vi "10-Tap 8-bit Camera with DRAM (FPGA).vi"() -> ()   [LabVIEW 2013]
doc: "This is the FPGA VI for the 10-Tap 8-Bit Camera with DRAM example. This example demonstrates how to acquire images from a 10-tap, 8-bit, extended configuration, Camera Link camera and transfer the images to the host. This example supports area scan and line scan cameras for both continuous and finite acquisitions.\n\nThis example also demonstrates the use of DRAM as a frame buffer for very high speed acquisitions. Data packing and flow-control are also employed to maximize use of the available DRAM and FIFOs in terms of both memory space and performance.\n\nAdditionally, the example demonstrates the serial server, which allows third-party camera configuration utilities to communicate with the camera using the Camera Link serial interface while this VI is running."
uses:
  Common/CL Signal Mapping.ctl
  Common/CL Configuration.ctl
  FPGA/Sector/Accumulate/Sector Parameter Cluster.ctl
  <vilib>/Platform/TimedLoop/XDataNode/timing_clust.ctl
  <vilib>/Platform/TimedLoop/XDataNode/nitl_modes.ctl
  <vilib>/Platform/TimedLoop/XDataNode/wakeup.ctl
  <vilib>/rvi/Emulation/niFpgaSctlEmulationGetInTimedLoop.vi
  <vilib>/rvi/Emulation/niFpgaEmulationReportErrorSimple.vi
  <vilib>/rvi/Emulation/niFpgaGetClockAttributes.vi
  <vilib>/rvi/Emulation/niFpgaCriticalErrorInLSC.vi
  <vilib>/rvi/eio/common/nirviEmuTemplateMethod_errors.vi
  FPGA/Globals/Wing Square Wave Frequency Global.vi
  <vilib>/rvi/interface/RandomDataEmulation/nirviRandomDataFPGAFIFO.vi
  <vilib>/rvi/interface/RandomDataEmulation/niFpgaRandomDataHandleErrors.vi
  <vilib>/rvi/FIFO/Fifo_Resource/nirvififoEmulationWriteFpgaImpl.vi
  <vilib>/rvi/DataTransferAndStorage/Container/Common/niFpgaContainerGetUniqueNameForEmu.vi
  <vilib>/rvi/FIFO/Fifo_Resource/nirvififoEmulationGetNumberOfElementsToReadFpgaImpl.vi
  <vilib>/rvi/FIFO/Fifo_Resource/nirvififoEmulationReadFpgaImpl.vi
  <vilib>/rvi/FIFO/Fifo_Resource/nirvififoEmulationGetNumberOfElementsToWriteFpgaImpl.vi
  <vilib>/rvi/Emulation/niFpgaProcessEmulError.vi
  FPGA/Globals/Sector Parameter Global.vi
  FPGA/Globals/Accumulated Sector Intensity.vi
  FPGA/Globals/Pixel Location Global.vi
  <vilib>/Platform/TimedLoop/XDataNode/XDataNode.xnode
  <vilib>/eio/EIONode/EIONode.xnode
  <vilib>/rvi/DataTransferAndStorage/Container/XNode/niFpgaContainer.xnode
  <vilib>/rvi/interface/RandomDataEmulation/nirviRandomDataFpgaReadWriteTemplate.vi
  <vilib>/rvi/FIFO/Fifo_Resource/nirvififoEmulationWrite.vi
  <vilib>/rvi/FIFO/Fifo_Resource/nirvififoEmulationGetNumberOfElementsToRead.vi
  <vilib>/rvi/FIFO/Fifo_Resource/nirvififoEmulationRead.vi
  <vilib>/rvi/FIFO/Fifo_Resource/nirvififoEmulationGetNumberOfElementsToWrite.vi
  <vilib>/Platform/TimedLoop/XDataNode/XDNodeRunTimeDep.lvlib
  Common/CL Data to Pixels/10 Tap 8-Bit.vi
  FPGA/10-Tap Data/10-Tap Conversion Enum.ctl
panel:
  in  "[Average BG Intensity]":u8[](array[numeric])=[0, 0, 0, 0, 0, 0, 0, 0, 0, 0, 0, 0, 0, 0, 0, 0, 0, 0, 0, 0, 0, 0, 0, 0, 0, 0, 0, 0, 0, 0, 0, 0]
  in  "Sector Threshold":u8
  in  "# of Frames to Average":u8
  in  "Sector Parameters Right":T1={"Start Angle"=0.0, "End Angle"=0.4708251953125, "Inner Radius"=309, "Outter Radius"=405, "Hinge X"=685, "Hinge Y"=527, "NumWingSectors"=8}
  in  "Sector Parameters Left":T1={"Start Angle"=0.65740966796875, "End Angle"=0.99468994140625, "Inner Radius"=309, "Outter Radius"=405, "Hinge X"=464, "Hinge Y"=534, "NumWingSectors"=8}
  in  "Sim":bool=TRUE
  in  "CL Config.Configuration":T2=enum."Full"
  in  "CL Config.Signal Mapping":T3=enum."Basler 10-tap"
  in  "CL Config.Line Scan":bool
  in  "CL Config.DVAL Active High":bool=TRUE
  in  "CL Config.LVAL Active High":bool=TRUE
  in  "CL Config.FVAL Active High":bool=TRUE
  in  "CL Config.Spare Active High":bool=TRUE
  in  "Acq Control.Line Scan Height":u32
  in  "Acq Control.Frames To Acq":u32
  in  "Acq Control.Acquire":bool
  in  "Acq Control.Cancel Acq":bool
  in  "Acq Control.Ignore DVAL":bool
  in  "Acq Control.Initialize":bool
  out "Acq Status.Acq In Progress":bool
  out "Acq Status.Clocks Per Line":u32
  out "Acq Status.Frames Acq'd":u32
  out "Acq Status.Lines Per Frame":u32
  out "Acq Status.DMA Write Timeout":bool
  out "Acq Status.Initialized":bool
  in  "UART.Baud Rate":u8
  in  "UART.Transmit":bool
  in  "UART.Tx Data":u8[](array[numeric])=[0, 0, 0, 0, 0, 0, 0, 0, 0, 0] format="%02x"
  in  "UART.Set Baud Rate":bool
  in  "UART.Byte Mode":bool=TRUE
  out "UART.Rx Ready":bool
  out "UART.Break Indicator":bool
  out "UART.Framing Error":bool
  out "UART.Overrun Error":bool
  out "UART.Tx Ready":bool
  out "UART.Rx Data":u8 format="%02x"
  in  "UART.Receive":bool
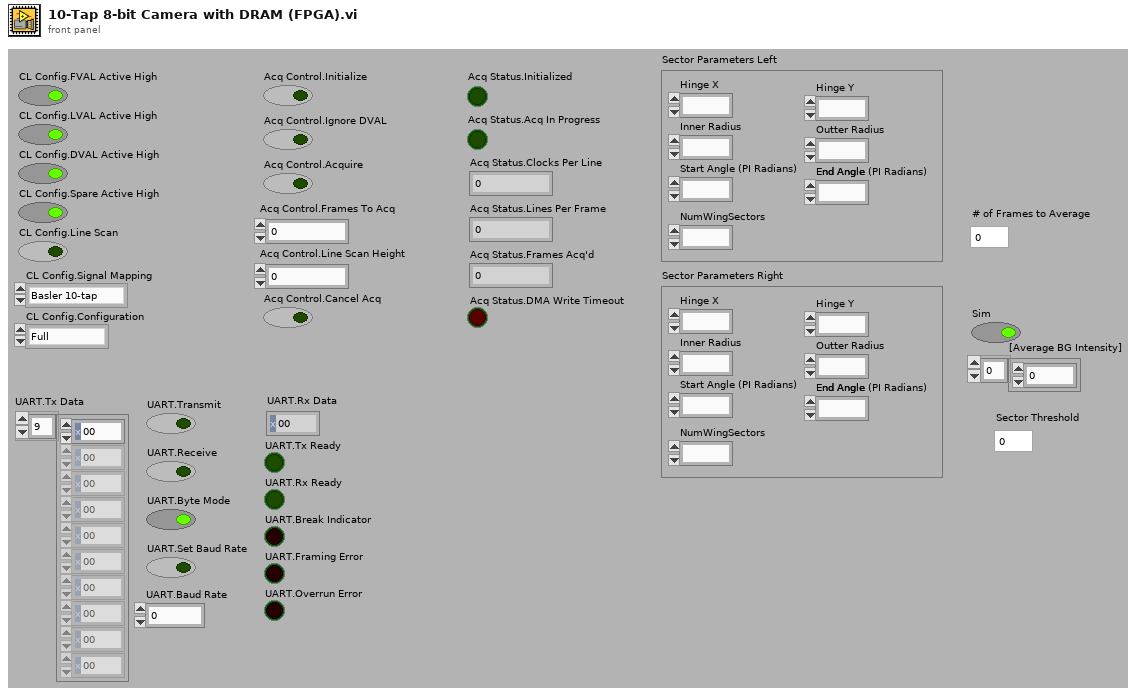
[diagram p1: front panel]
types:
  T1 = typedef "Sector Parameter Cluster.ctl" = cluster{"Start Angle":fxp<+/-,17,2>, "End Angle":fxp<+,17,3>, "Inner Radius":u16, "Outter Radius":u16, "Hinge X":u16, "Hinge Y":u16, "NumWingSectors":u8}
  T2 = typedef "CL Configuration.ctl" = enum8{"Base", "Medium", "Full"}
  T3 = typedef "CL Signal Mapping.ctl" = enum8{"Standard", "Basler 10-tap", "Vosskühler 10-tap"}
  T4 = typedef "XDNodeRunTimeDep.lvlib/timing_clust.ctl" = cluster{"Expected End [f-1]":u64, "Actual End [f-1]":u64, "Finished Late? [f-1]":bool, "Expected End [i-1]":u64, "Actual End [i-1]":u64, "Finished Late? [i-1]":bool, "Expected Start [i]":u64, "Actual Start [i]":u64, "Expected Start [f]":u64, "Actual Start [f]":u64, "Source Name":string, "Structure Name":string, "Period":i64, "Deadline":i64, "Offset":i64, "Start":i64, "Priority":i32, "Timeout":i32, "Mode":T5, "Wakeup Reason":T6, "Error":errorcluster, "Source Type":string, "Secondary Source Type":string, "Global End Time":u64, "Global Start Time":u64, "Frame Duration":u64, "Iteration Duration":u64, "Assigned CPU":i32, "I/O Scan Engine Mode":u32}
  T5 = typedef "XDNodeRunTimeDep.lvlib/nitl_modes.ctl" = enum32{"No Change", "Process missed periods, maintain original phase", "Discard missed periods, maintain original phase", "Process missed periods, ignore original phase", "Discard missed periods, ignore original phase"}
  T6 = typedef "XDNodeRunTimeDep.lvlib/wakeup.ctl" = enum32{"Normal", "Aborted", "Asynchronous wakeup", "Timing source error", "Timed loop error", "Timeout"}
  T7 = typedef "10-Tap Conversion Enum.ctl" = enum16{"10-Tap to 16 and 64", "16 and 64 to 10-Tap"}
  T8 = cluster{"Enables Valid":bool, "Frame Valid":bool, "Line Valid":bool, "Data Valid":bool}
  T9 = typedef "10-Tap 8-bit Cluster.ctl" = cluster{"Pixel 0":u8, "Pixel 1":u8, "Pixel 2":u8, "Pixel 3":u8, "Pixel 4":u8, "Pixel 5":u8, "Pixel 6":u8, "Pixel 7":u8, "Pixel 8":u8, "Pixel 9":u8}
  T10 = typedef "Image Type" = u32
  T11 = typedef "IMAQ Image.ctl" = refnum<image>
  T12 = cluster{"Tx Data":u8[], "Transmit":bool, "Receive":bool, "Byte Mode":bool, "Set Baud Rate":bool, "Baud Rate":u8}
  T13 = cluster{"Rx Data":u8, "Turn Off Transmit":bool, "Turn Off Receive":bool, "Turn Off Set Baud Rate":bool, "Tx Ready":bool, "Rx Ready":bool, "Break Indicator":bool, "Framing Error":bool, "Overrun Error":bool}
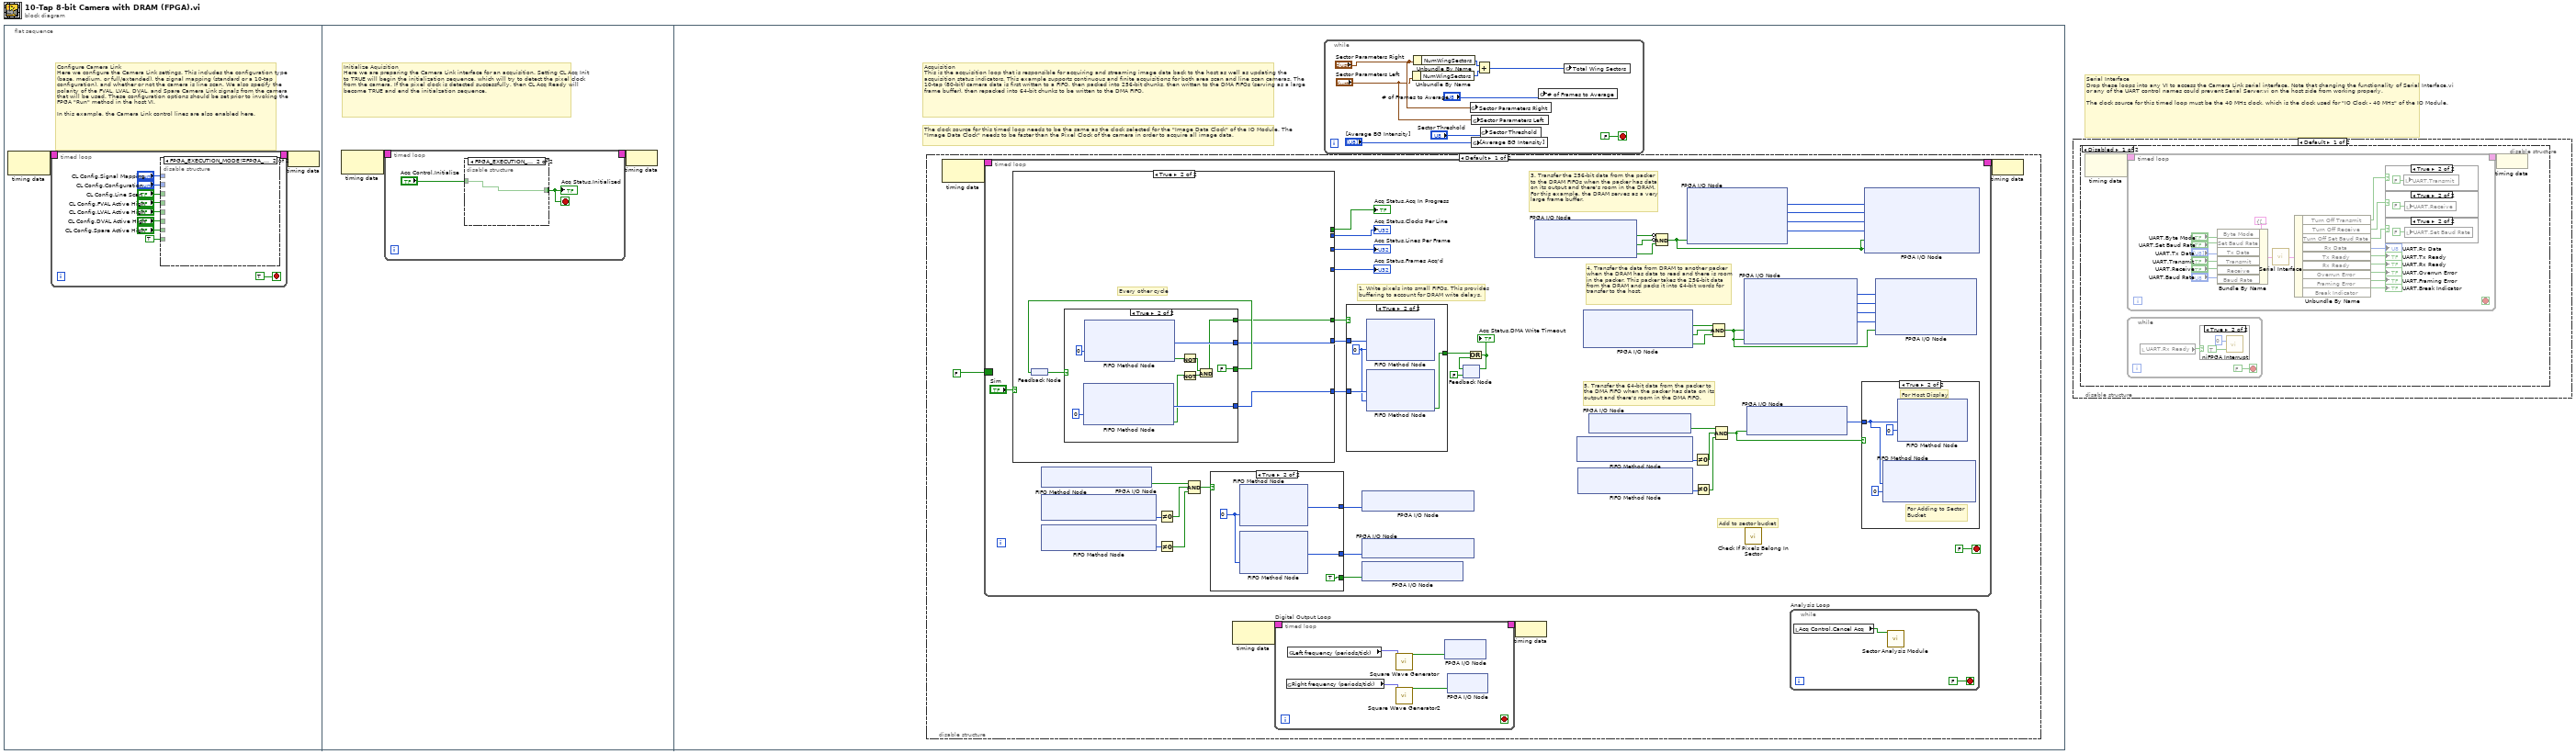
[diagram p0: block diagram]
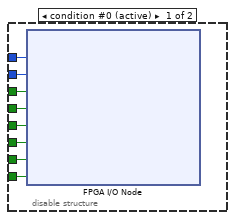
[diagram p8: hidden frame]
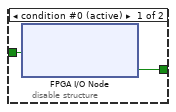
[diagram p9: hidden frame]
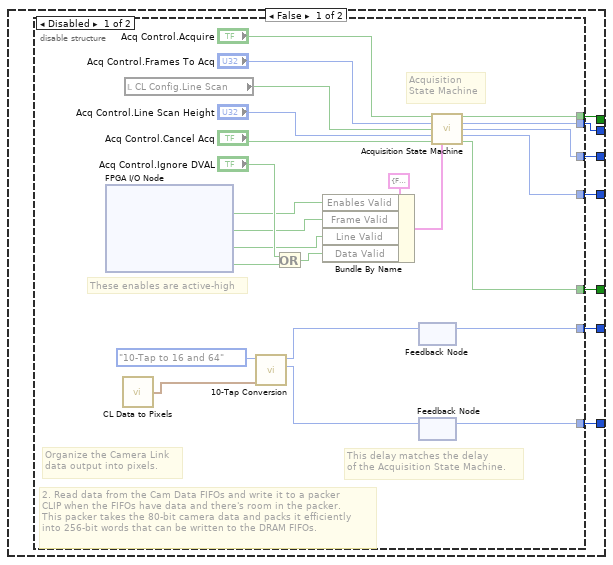
[diagram p11: hidden frame]
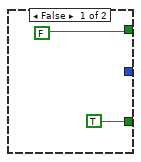
[diagram p13: hidden frame]
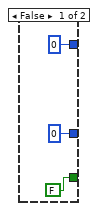
[diagram p14: hidden frame]
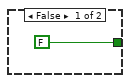
[diagram p15: hidden frame]
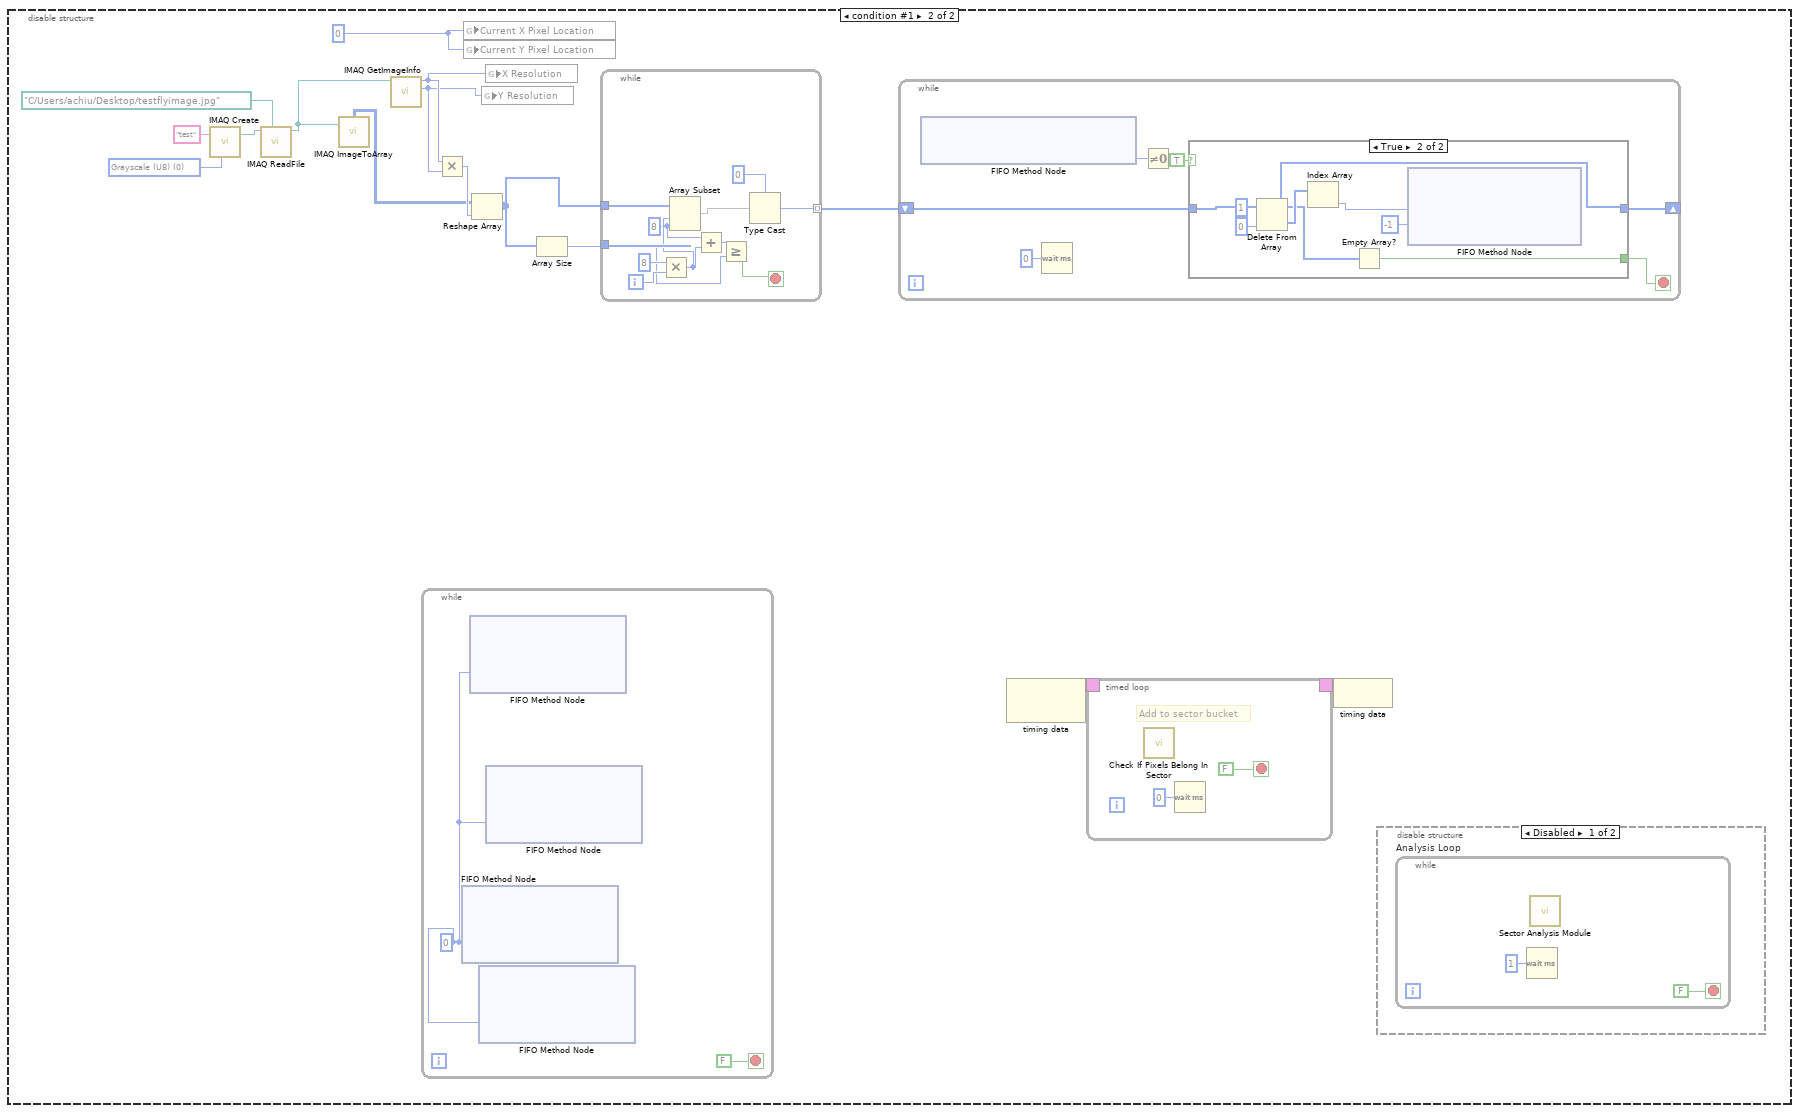
[diagram p16: hidden frame]
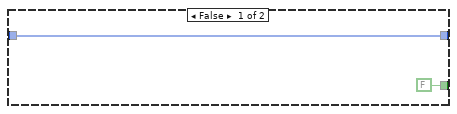
[diagram p18: hidden frame]
diagram:
  # "Serial Interface\nDrop these loops into any VI to access the Camera Link serial interface. Note that changing the functionality of Serial Interface.vi or any of the UART control names could prevent Serial Server.vi on the host side from working properly.\n\nThe clock source for this timed loop must be the 40 MHz clock, which is the clock used for \"IO Clock - 40 MHz\" of the IO Module."
  n1 = flat-sequence {
    frame #0 {
      # "Configure Camera Link\nHere we configure the Camera Link settings. This includes the configuration type (base, medium, or full/extended), the signal mapping (standard or a 10-tap configuration), and whether or not the camera is line scan. We also specify the polarity of the FVAL, LVAL, DVAL, and Spare Camera Link signals from the camera that will be used. These configuration options should be set prior to invoking the FPGA \"Run\" method in the host VI.\n\nIn this example, the Camera Link control lines are also enabled here."
      n2 = node-c288() -> (w2:T4)  [unwired: 1 in]
      n3 = timed-loop {
        timing: w2 -> [_]
        timing-out: [_] -> w1
        stop <- TRUE stop-if-true
        n4 = disable-structure shown="FPGA_EXECUTION_MODE!=FPGA_TARGET" {
          disable-tunnel: "CL Config.FVAL Active High" -> [w19 _]
          disable-tunnel: "CL Config.LVAL Active High" -> [w18 _]
          disable-tunnel: "CL Config.DVAL Active High" -> [w17 _]
          disable-tunnel: "CL Config.Spare Active High" -> [w16 _]
          disable-tunnel: "CL Config.Signal Mapping" -> [w15 _]
          disable-tunnel: "CL Config.Configuration" -> [w14 _]
          disable-tunnel: "CL Config.Line Scan" -> [w13 _]
          disable-tunnel: TRUE ("IO Module\\CL Control Enable") -> [w12 _]
          frame condition #0 (active) {
            n5 = xnode "FPGA I/O Node"("CL Set Signal Mapping"=w15, "CL Set Configuration"=w14, "CL Set Line Scan"=w13, "CL Set FVAL Active High"=w19, "CL Set LVAL Active High"=w18, "CL Set DVAL Active High"=w17, "CL Set Spare Active High"=w16, "CL Control Enable"=w12) -> ()  [unwired: 8 in, 8 out]
          }
          frame condition #1 {
          }
        }
      }
      n6 = node-c288(w1) -> ()
    }
    frame #1 {
      # "Initialize Aquisition\nHere we are preparing the Camera Link interface for an acquisition. Setting CL Acq Init to TRUE will begin the initialization sequence, which will try to detect the pixel clock from the camera. If the pixel clock is detected successfully, then CL Acq Ready will become TRUE and end the initialzation sequence."
      n7 = node-c288() -> (w25:T4)  [unwired: 1 out]
      n8 = timed-loop {
        timing: w25 -> [_]
        timing-out: [_] -> w24
        stop <- w26 stop-if-true
        n9 = disable-structure shown="FPGA_EXECUTION_MODE!=FPGA_TARGET" {
          disable-tunnel: "Acq Control.Initialize" -> [w29 w30]
          disable-tunnel: [w28 w30] -> w26
          frame condition #0 (active) {
            n10 = xnode "FPGA I/O Node"("CL Acq Init"=w29) -> ("CL Acq Ready"=w28:bool)  [unwired: 2 in, 2 out]
          }
          frame condition #1 {
          }
        }
        "Acq Status.Initialized" <- w26
      }
      n11 = node-c288(w24) -> ()
    }
    frame #2 {
      # "The clock source for this timed loop needs to be the same as the clock selected for the \"Image Data Clock\" of the IO Module. The \"Image Data Clock\" needs to be faster than the Pixel Clock of the camera in order to acquire all image data."
      # "Acquisition\nThis is the acquisition loop that is responsible for acquiring and streaming image data back to the host as well as updating the acquisition status indicators. This example supports continuous and finite acquisitions for both area scan and line scan cameras. The 10-tap (80-bit) camera data is first written to a FIFO, then packed into 256-bit chunks, then written to the DMA FIFOs (serving as a large frame buffer), then repacked into 64-bit chunks to be written to the DMA FIFO."
      n12 = disable-structure shown="Default" {
        frame condition #0 (active) {
          n13 = node-c288() -> (w48:T4)  [unwired: 1 in]
          n14 = timed-loop {
            timing: w48 -> [_]
            timing-out: [_] -> w47
            border: FALSE -> [_]
            stop <- FALSE stop-if-true
            # "Add to sector bucket"
            # "5. Transfer the 64-bit data from the packer to\nthe DMA FIFO when the packer has data on its\noutput and there's room in the DMA FIFO."
            # "4. Transfer the data from DRAM to another packer\nwhen the DRAM has data to read and there is room\nin the packer. This packer takes the 256-bit data\nfrom the DRAM and packs it into 64-bit words for\ntransfer to the host."
            # "3. Transfer the 256-bit data from the packer\nto the DRAM FIFOs when the packer has data\non its output and there's room in the DRAM.\nFor this example, the DRAM serves as a very\nlarge frame buffer."
            # "1. Write pixels into small FIFOs. This provides\nbuffering to account for DRAM write delays."
            n15 = case shown="True" "Sim" {
              tunnel: [w112 w137] -> w102
              tunnel: [w111 w138] -> w97
              tunnel: [w106 w140] -> w85
              tunnel: [w110 _] -> w84
              tunnel: [w109 _] -> w83
              tunnel: [w108 _] -> w82
              tunnel: [w107 _] -> w81
              frame False {
                n16 = disable-structure shown="Disabled" {
                  disable-tunnel: [w136 _] -> w112
                  disable-tunnel: [w135 _] -> w111
                  disable-tunnel: [w121 _] -> w110
                  disable-tunnel: [w120 _] -> w109
                  disable-tunnel: [w119 _] -> w108
                  disable-tunnel: [w118 _] -> w107
                  disable-tunnel: [w117 _] -> w106
                  frame Disabled {
                    # "These enables are active-high"
                    # "Acquisition\nState Machine"
                    # "2. Read data from the Cam Data FIFOs and write it to a packer\nCLIP when the FIFOs have data and there's room in the packer.\nThis packer takes the 80-bit camera data and packs it efficiently\ninto 256-bit words that can be written to the DRAM FIFOs."
                    # "Organize the Camera Link\ndata output into pixels."
                    # "This delay matches the delay\nof the Acquisition State Machine."
                    n17 = xnode "FPGA I/O Node"() -> ("CL Output Valid"=w125:bool, "CL Frame Valid"=w126:bool, "CL Line Valid"=w127:bool, "CL Data Valid"=w130:bool)  [unwired: 4 in, 4 out]
                    n18 = call-poly "CL Data to Pixels.vi"() -> ("Pixels"=w113:T9)  [unwired: 1 in]
                    n19 = local read "CL Config.Line Scan"() -> (w133:bool)
                    n20 = call "10-Tap Conversion.vi"("10 Tap In"=w113, "Operation"=10-Tap_Conversion_Enum."10-Tap to 16 and 64") -> ("64 Bit Out"=w114:u64, "16 Bit Out"=w115:u16)  [unwired: 7 in, 1 out]
                    n21 = Or(x="Acq Control.Ignore DVAL", y=w130) -> (x .or. y?=w131:bool)
                    n22 = Bundle By Name(cluster=T8 {"Enables Valid"=FALSE, "Frame Valid"=FALSE, "Line Valid"=FALSE, "Data Valid"=FALSE} ("Enables"), "Enables Valid"=w125, "Frame Valid"=w126, "Line Valid"=w127, "Data Valid"=w131) -> (w128:T8)
                    n23 = feedback #1() -> (w135:u16)  [unwired: 1 in]
                    n24 = feedback-in #1(w115) -> ()
                    n25 = feedback #2() -> (w136:u64)  [unwired: 1 in]
                    n26 = feedback-in #2(w114) -> ()
                    n27 = call "Acquisition State Machine.vi"("Acquire"="Acq Control.Acquire", "Frames to Acquire"="Acq Control.Frames To Acq", "Line Scan"=w133, "Line Scan Height"="Acq Control.Line Scan Height", "Cancel Acq"="Acq Control.Cancel Acq", "Enables"=w128) -> ("Acq In Progress"=w121:bool, "Num Clocks Per Line"=w120:u32, "Num Lines Per Frame"=w119:u32, "Num Frames Acq'd"=w118:u32, "Capture Cycle"=w117:bool)  [unwired: 4 in, 1 out]
                  }
                  frame Enabled {
                  }
                }
              }
              frame True {
                # "Every other cycle"
                n28 = feedback #3() -> (w139:bool)
                n29 = case shown="True" w139 {
                  tunnel: [_ w153] -> w138
                  tunnel: [_ w152] -> w137
                  tunnel: [FALSE w145] -> w140
                  tunnel: [TRUE FALSE] -> w141
                  frame False {
                  }
                  frame True {
                    n30 = xnode ("FIFO Method Node")("Timeout"=0) -> ("Element"=w152:u64, "Timed Out?"=w148:bool)  [unwired: 1 in, 1 out]
                    n31 = xnode ("FIFO Method Node")("Timeout"=0) -> ("Element"=w153:u16, "Timed Out?"=w149:bool)  [unwired: 1 in, 1 out]
                    n32 = Not(x=w149) -> (.not. x?=w147:bool)
                    n33 = Not(x=w148) -> (.not. x?=w146:bool)
                    n34 = And(x=w147, y=w146) -> (x .and. y?=w145:bool)
                  }
                }
                n35 = feedback-in #3(w141) -> ()
              }
            }
            "Acq Status.Frames Acq'd" <- w81
            "Acq Status.Lines Per Frame" <- w82
            "Acq Status.Clocks Per Line" <- w83
            "Acq Status.Acq In Progress" <- w84
            n36 = xnode "FPGA I/O Node"() -> ("Pack 80 to 256\\Ready For Write"=w91:bool)  [unwired: 1 in, 1 out]
            n37 = xnode ("FIFO Method Node")() -> ("Number of Elements to Read"=w95:u32)  [unwired: 1 in, 1 out]
            n38 = xnode ("FIFO Method Node")() -> ("Number of Elements to Read"=w94:u32)  [unwired: 1 in, 1 out]
            n39 = Not Equal To 0?(x=w95) -> (x != 0?=w89:bool)
            n40 = Not Equal To 0?(x=w94) -> (x != 0?=w88:bool)
            n41 = Compound Arithmetic op=AND(w91, w89, w88) -> (w90:bool)
            n42 = case shown="True" w90 {
              tunnel: [u16 0 ("Element") w160] -> w96
              tunnel: [u64 0 ("Element") w159] -> w92
              tunnel: [FALSE TRUE] -> w93
              frame False {
              }
              frame True {
                w158 = 0 ("Timeout")
                n43 = xnode ("FIFO Method Node")("Timeout"=w158) -> ("Element"=w160:u16)  [unwired: 1 in, 2 out]
                n44 = xnode ("FIFO Method Node")("Timeout"=w158) -> ("Element"=w159:u64)  [unwired: 1 in, 2 out]
              }
            }
            n45 = case shown="True" w85 {
              tunnel: [FALSE ("Timed Out?") w164] -> w100
              tunnel: w102 -> [_ w165]
              tunnel: w97 -> [_ w163]
              frame False {
              }
              frame True {
                w162 = 0 ("Timeout")
                n46 = xnode ("FIFO Method Node")("Element"=w163, "Timeout"=w162) -> ()  [unwired: 1 in, 2 out]
                n47 = xnode ("FIFO Method Node")("Element"=w165, "Timeout"=w162) -> ("Timed Out?"=w164:bool)  [unwired: 1 in, 1 out]
              }
            }
            n48 = xnode "FPGA I/O Node"("Pack 80 to 256\\Data In Upper 16"=w96) -> ()  [unwired: 1 in, 1 out]
            n49 = xnode "FPGA I/O Node"("Pack 80 to 256\\Data In Lower 64"=w92) -> ()  [unwired: 1 in, 1 out]
            n50 = xnode "FPGA I/O Node"("Pack 80 to 256\\Write Enable"=w93) -> ()  [unwired: 1 in, 1 out]
            n51 = feedback #4(FALSE) -> (w99:bool)
            n52 = Or(x=w100, y=w99) -> (x .or. y?=w98:bool)
            "Acq Status.DMA Write Timeout" <- w98
            n53 = feedback-in #4(w98) -> ()
            n54 = xnode "FPGA I/O Node"() -> ("DRAM Bank 0\\Full"=w61:bool, "Pack 80 to 256\\Output Valid"=w80:bool)  [unwired: 3 in, 4 out]
            n55 = xnode ("FIFO Method Node")() -> ("Number of Elements to Write"=w63:u32)  [unwired: 1 in, 1 out]
            n56 = xnode ("FIFO Method Node")() -> ("Number of Elements to Write"=w60:u32)  [unwired: 1 in, 1 out]
            n57 = xnode "FPGA I/O Node"() -> ("DRAM Bank 1\\Data_Available"=w74:bool, "DRAM Bank 0\\Data_Available"=w72:bool, "Pack 256 to 64\\Ready for Write"=w73:bool)  [unwired: 3 in, 3 out]
            n58 = xnode "FPGA I/O Node"() -> ("Pack 256 to 64\\Output Valid"=w65:bool)  [unwired: 1 in, 1 out]
            n59 = Compound Arithmetic op=AND(invert w61, invert w61, w80) -> (w75:bool)
            n60 = xnode "FPGA I/O Node"("Pack 80 to 256\\Read Enable"=w75) -> ("Pack 80 to 256\\Data Out 3"=w79:u64, "Pack 80 to 256\\Data Out 2"=w78:u64, "Pack 80 to 256\\Data Out 1"=w77:u64, "Pack 80 to 256\\Data Out 0"=w76:u64)  [unwired: 5 in, 5 out]
            n61 = Not Equal To 0?(x=w63) -> (x != 0?=w64:bool)
            n62 = Not Equal To 0?(x=w60) -> (x != 0?=w59:bool)
            n63 = Compound Arithmetic op=AND(w74, w72, w73) -> (w67:bool)
            n64 = Compound Arithmetic op=AND(w65, w64, w59) -> (w62:bool)
            n65 = xnode "FPGA I/O Node"("DRAM Bank 1\\Read"=w67, "DRAM Bank 0\\Read"=w67) -> ("DRAM Bank 1\\Read_Data_Upper"=w71:u64, "DRAM Bank 1\\Read_Data_Lower"=w70:u64, "DRAM Bank 0\\Read_Data_Upper"=w69:u64, "DRAM Bank 0\\Read_Data_Lower"=w68:u64)  [unwired: 6 in, 6 out]
            n66 = call "Check If Pixels Belong In Sector.vi"() -> ()  [unwired: 11 in, 1 out]
            n67 = xnode "FPGA I/O Node"("Pack 256 to 64\\Read Enable"=w62) -> ("Pack 256 to 64\\Data Out 64"=w66:u64)  [unwired: 2 in, 2 out]
            n68 = case shown="True" w62 {
              tunnel: w66 -> [_ w104]
              frame False {
              }
              frame True {
                # "For Adding to Sector \nBucket"
                # "For Host Display"
                n69 = xnode ("FIFO Method Node")("Element"=w104, "Timeout"=0) -> ()  [unwired: 1 in, 2 out]
                n70 = xnode ("FIFO Method Node")("Element"=w104, "Timeout"=0) -> ()  [unwired: 1 in, 2 out]
              }
            }
            n71 = xnode "FPGA I/O Node"("DRAM Bank 1\\Write_Data_Upper"=w79, "DRAM Bank 1\\Write_Data_Lower"=w78, "DRAM Bank 0\\Write_Data_Upper"=w77, "DRAM Bank 0\\Write_Data_Lower"=w76, "DRAM Bank 1\\Write"=w75, "DRAM Bank 0\\Write"=w75) -> ()  [unwired: 6 in, 6 out]
            n72 = xnode "FPGA I/O Node"("Pack 256 to 64\\Data In 3"=w71, "Pack 256 to 64\\Data In 2"=w70, "Pack 256 to 64\\Data In 1"=w69, "Pack 256 to 64\\Data In 0"=w68, "Pack 256 to 64\\Write Enable"=w67) -> ()  [unwired: 5 in, 5 out]
          }
          n73 = node-c288() -> (w46:T4)  [unwired: 1 in]
          n74 = timed-loop "Digital Output Loop" {
            timing: w46 -> [_]
            timing-out: [_] -> w45
            stop <- _ stop-if-true
            n75 = global read "Wing Square Wave Frequency Global.vi" "Right frequency (periods/tick)"() -> (w51:fxp<+,32,0>)
            n76 = global read "Wing Square Wave Frequency Global.vi" "Left frequency (periods/tick)"() -> (w52:fxp<+,32,0>)
            n77 = call "Square Wave Generator"("frequency (periods/tick)"=w52) -> ("square wave out"=w54:bool)  [unwired: 14 in]
            n78 = call "Square Wave Generator2"("frequency (periods/tick)"=w51) -> ("square wave out"=w53:bool)  [unwired: 14 in]
            n79 = xnode "FPGA I/O Node"("TTL 0"=w54) -> ()  [unwired: 1 in, 1 out]
            n80 = xnode "FPGA I/O Node"("TTL 1"=w53) -> ()  [unwired: 1 in, 1 out]
          }
          n81 = node-c288(w45) -> ()
          n82 = while "Analysis Loop" {
            stop <- FALSE stop-if-true
            n83 = local read "Acq Control.Cancel Acq"() -> (w49:bool)
            n84 = call "Sector Analysis Module.vi"("Canceled?"=w49) -> ()  [unwired: 8 in, 3 out]
          }
          n85 = node-c288(w47) -> ()
        }
        frame condition #1 {
          w180 = u16 0 ("Current X Pixel Location")
          w183 = T10 0 items=["Grayscale (U8)", "Grayscale (I16)", "Grayscale (SGL)", "Complex (CSG)", "RGB (U32)", "HSL (U32)", "RGB (U64)", "Grayscale (U16)"] ("Image Type")
          n86 = call "IMAQ Create"("Image Name"="test", "Image Type"=w183) -> ("New Image"=w182:T11)  [unwired: 3 in, 1 out]
          n87 = call "IMAQ ReadFile"("File Path"=path "C:/Users/achiu/Desktop/testflyimage.jpg", "Image"=w182) -> ("Image Out"=w172:T11)  [unwired: 5 in, 4 out]
          n88 = call "IMAQ ImageToArray"("Image"=w172) -> ("Image Pixels (U8)"=w176:u8[][])  [unwired: 3 in, 4 out]
          n89 = call "IMAQ GetImageInfo"("Image"=w172) -> ("Y Resolution"=w173:i32, "X Resolution"=w174:i32)  [unwired: 3 in, 6 out]
          n90 = while {
            stop <- FALSE stop-if-true
            w187 = 0 ("Timeout")
            n91 = xnode ("FIFO Method Node")("Timeout"=w187) -> ()  [unwired: 1 in, 3 out]
            n92 = xnode ("FIFO Method Node")("Timeout"=w187) -> ()  [unwired: 1 in, 3 out]
            n93 = xnode ("FIFO Method Node")("Timeout"=w187) -> ()  [unwired: 1 in, 3 out]
            n94 = xnode ("FIFO Method Node")("Timeout"=w187) -> ()  [unwired: 1 in, 3 out]
          }
          n95 = Multiply(x=w174, y=w173) -> (x*y=w177:i32)
          n96 = global write "Pixel Location Global.vi" "Current X Pixel Location"(w180) -> ()
          n97 = global write "Pixel Location Global.vi" "Current Y Pixel Location"(w180) -> ()
          n98 = Reshape Array(w176, w177) -> (w178:u8[])
          n99 = global write "Pixel Location Global.vi" "Y Resolution"(w173) -> ()
          n100 = global write "Pixel Location Global.vi" "X Resolution"(w174) -> ()
          n101 = Array Size(array=w178) -> (size(s)=w179:i32)
          n102 = while {
            tunnel: w179 -> [w215]
            tunnel: w178 -> [w219]
            tunnel: [w211] -> w175 mode=indexing
            i -> [w221]
            stop <- w214 stop-if-true
            w217 = 8 ("length")
            n103 = Multiply(x=8, y=w221) -> (x*y=w218:i32)
            n104 = Array Subset(array=w219, index=w218, length=w217) -> (w213:u8[])
            n105 = Add(x=w217, y=w218) -> (x+y=w216:i32)
            n106 = Greater Or Equal?(x=w216, y=w215) -> (x >= y?=w214:bool)
            n107 = Type Cast(type=u64 0, x=w213) -> (*(type *) &x=w211:u64)
          }
          n108 = while {
            shift-right: [w191] -> _
            shift-left: w175 -> [w194]
            stop <- w192 stop-if-true
            n109 = xnode ("FIFO Method Node")() -> ("Number of Elements to Write"=w193:u32)  [unwired: 1 in, 1 out]
            n110 = Wait (ms)(milliseconds to wait=u32 0) -> ()  [unwired: 1 out]
            n111 = Not Equal To 0?(x=w193) -> ()  [unwired: 1 out]
            n112 = case shown="True" TRUE {
              tunnel: w194 -> [w195 w204]
              tunnel: [FALSE ("empty?") w198] -> w192
              tunnel: [w195 w197] -> w191
              frame False {
              }
              frame True {
                n113 = Delete From Array(array=w204, length=1, index=0) -> (deleted portion=w199:u64[], array with subset deleted=w197:u64[])
                n114 = Index Array(array=w199) -> (element=w200:u64)  [unwired: 1 in]
                n115 = Empty Array?(array=w197) -> (empty?=w198:bool)
                n116 = xnode ("FIFO Method Node")("Element"=w200, "Timeout"=-1) -> ()  [unwired: 1 in, 2 out]
              }
            }
          }
          n117 = node-c288() -> (w171:T4)  [unwired: 1 in]
          n118 = timed-loop {
            timing: w171 -> [_]
            timing-out: [_] -> w170
            stop <- FALSE stop-if-true
            # "Add to sector bucket"
            n119 = call "Check If Pixels Belong In Sector.vi"() -> ()  [unwired: 11 in, 1 out]
            n120 = Wait (ms)(milliseconds to wait=u32 0) -> ()  [unwired: 1 out]
          }
          n121 = node-c288(w170) -> ()
          n122 = disable-structure shown="Disabled" {
            frame Disabled {
              n123 = while "Analysis Loop" {
                stop <- FALSE stop-if-true
                n124 = Wait (ms)(milliseconds to wait=u32 1) -> ()  [unwired: 1 out]
                n125 = call "Sector Analysis Module.vi"() -> ()  [unwired: 9 in, 3 out]
              }
            }
            frame Enabled {
            }
          }
        }
      }
      n126 = while {
        stop <- FALSE stop-if-true
        n127 = Unbundle By Name("Sector Parameters Left") -> ("NumWingSectors"=w41:u8)
        n128 = Unbundle By Name("Sector Parameters Right") -> ("NumWingSectors"=w42:u8)
        n129 = global write "Sector Parameter Global.vi" "Sector Parameters Right"("Sector Parameters Right") -> ()
        n130 = global write "Sector Parameter Global.vi" "Sector Parameters Left"("Sector Parameters Left") -> ()
        n131 = global write "Sector Parameter Global.vi" "[Average BG Intensity]"("[Average BG Intensity]") -> ()
        n132 = Add(x=w42, y=w41) -> (x+y=w40:u8)
        n133 = global write "Sector Parameter Global.vi" "Sector Threshold"("Sector Threshold") -> ()
        n134 = global write "Pixel Location Global.vi" "# of Frames to Average"("# of Frames to Average") -> ()
        n135 = global write "Accumulated Sector Intensity.vi" "Total Wing Sectors"(w40) -> ()
      }
    }
  }
  n136 = disable-structure shown="Default" {
    frame condition #0 (active) {
      n137 = disable-structure shown="Disabled" {
        frame Disabled {
          n138 = node-c288() -> (w223:T4)  [unwired: 1 out]
          n139 = timed-loop {
            timing: w223 -> [_]
            timing-out: [_] -> w222
            stop <- _ stop-if-true
            n140 = Bundle By Name(cluster=T12 {"Tx Data"=[0, 0, 0, 0, 0, 0, 0, 0, 0, 0], "Transmit"=FALSE, "Receive"=FALSE, "Byte Mode"=TRUE, "Set Baud Rate"=FALSE, "Baud Rate"=0} ("UART Inputs"), "Byte Mode"="UART.Byte Mode", "Set Baud Rate"="UART.Set Baud Rate", "Tx Data"="UART.Tx Data", "Transmit"="UART.Transmit", "Receive"="UART.Receive", "Baud Rate"="UART.Baud Rate") -> (w228:T12)
            n141 = call "Serial Interface.vi"("UART Inputs"=w228) -> ("UART Outputs"=w240:T13)
            n142 = Unbundle By Name(w240) -> ("Turn Off Transmit"=w233:bool, "Turn Off Receive"=w234:bool, "Turn Off Set Baud Rate"=w230:bool, "Rx Data"=→"UART.Rx Data":u8, "Tx Ready"=→"UART.Tx Ready":bool, "Rx Ready"=→"UART.Rx Ready":bool, "Overrun Error"=→"UART.Overrun Error":bool, "Framing Error"=→"UART.Framing Error":bool, "Break Indicator"=→"UART.Break Indicator":bool)
            n143 = case shown="True" w233 {
              frame False {
              }
              frame True {
                n144 = local write "UART.Transmit"(FALSE ("UART.Transmit")) -> ()
              }
            }
            n145 = case shown="True" w234 {
              frame False {
              }
              frame True {
                n146 = local write "UART.Receive"(FALSE ("UART.Receive")) -> ()
              }
            }
            n147 = case shown="True" w230 {
              frame False {
              }
              frame True {
                n148 = local write "UART.Set Baud Rate"(FALSE ("UART.Receive")) -> ()
              }
            }
          }
          n149 = while {
            stop <- FALSE stop-if-true
            n150 = local read "UART.Rx Ready"() -> (w225:bool)
            n151 = case shown="True" w225 {
              frame False {
              }
              frame True {
                n152 = call <vilib>:"niFPGA Interrupt.vi"("Wait Until Cleared (F)"=TRUE ("Wait Until Cleared"), "IRQ Number (0)"=u8 0 ("IRQ Number")) -> ()  [unwired: 1 in]
              }
            }
          }
          n153 = node-c288(w222) -> ()
        }
        frame Enabled {
        }
      }
    }
    frame condition #1 {
    }
  }
